vi "Save image.vi"(6 "Show filename dialog?":bool=TRUE, 7 "Extension (.tif)":string(combo)=".tif", 8 "error in":errorcluster, 9 "File name":string="image.tif", 10 "Image":T1, 11 "Base dir":path) -> (0 "error out":errorcluster, 3 "dup file":path)   [LabVIEW 2013, in "FileIO lib.lvlib"]
doc: "Creates a file and saves the current image. Image type is determined by the extension of the file name."
uses:
  FileIO lib.lvlib
  <vilib>/vision/Image Controls.llb/IMAQ Image.ctl
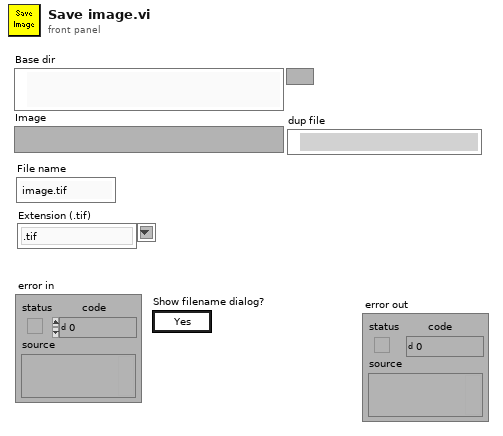
[diagram p1: front panel]
types:
  T1 = typedef "IMAQ Image.ctl" = refnum<image>
  T2 = enum32{"existing file", "new file", "new or existing file", "existing dir", "new dir", "new or existing dir", "existing file (use LLBs)", "new file (use LLBs)", "new or existing file (use LLBs)", "new or existing file or directory (use LLBs)"}
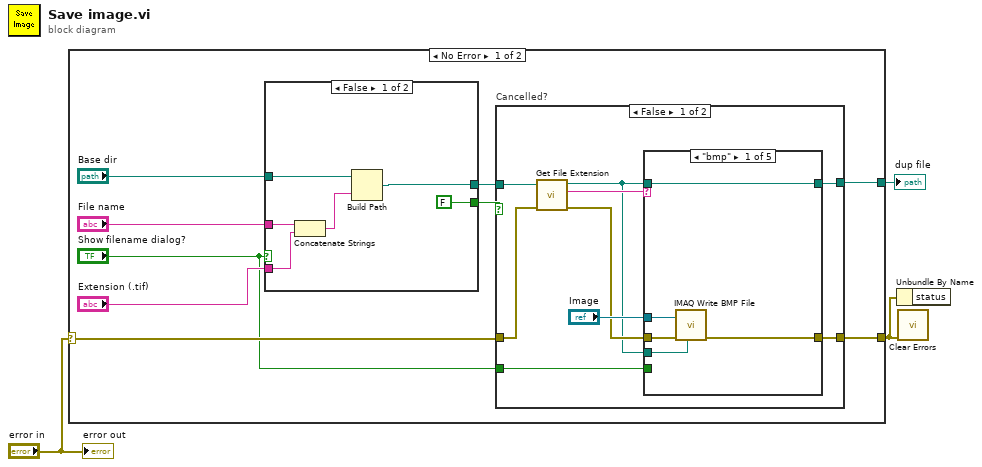
[diagram p0: block diagram]
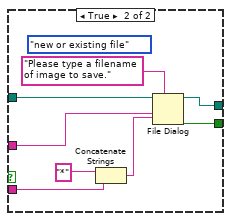
[diagram p2: hidden frame]
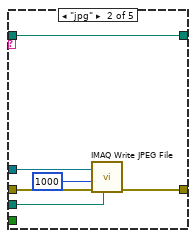
[diagram p3: hidden frame]
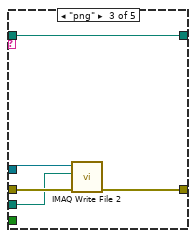
[diagram p4: hidden frame]
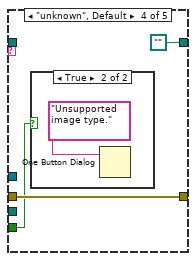
[diagram p5: hidden frame]
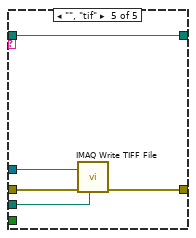
[diagram p7: hidden frame]
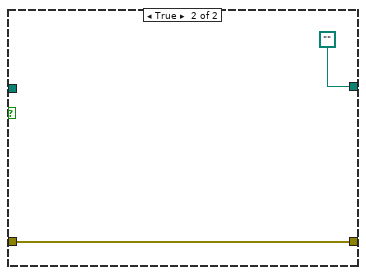
[diagram p8: hidden frame]
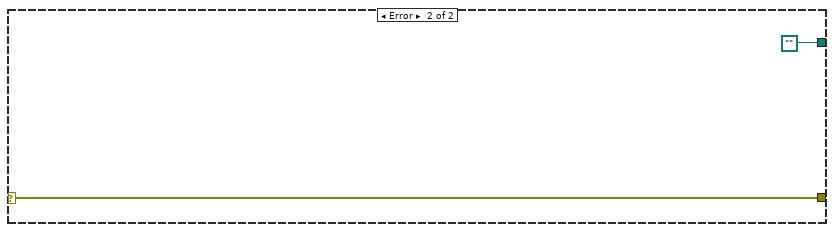
[diagram p9: hidden frame]
diagram:
  n1 = case shown="No Error" "error in" {
    selector: "error in" -> [w9 w64]
    tunnel: [w5 w64] -> w2
    tunnel: [w4 path ""] -> w1
    frame No Error {
      n2 = case shown="False" "Show filename dialog?" {
        tunnel: [w13 w26] -> w12
        tunnel: [FALSE ("cancelled") w25] -> w11
        tunnel: "Base dir" -> [w17 w23]
        tunnel: "File name" -> [w16 w22]
        tunnel: "Extension (.tif)" -> [w15 w20]
        frame False {
          n3 = Concatenate Strings(w16, w15) -> (w14:string)
          n4 = Build Path(base path=w17, name or relative path=w14) -> (appended path=w13:path)
        }
        frame True {
          (unwired) T2."new or existing file" ("select mode (2)")
          n5 = Concatenate Strings("*" ("pattern label"), w20) -> (w19:string)
          n6 = File Dialog(6:w19, 7:"Please type a filename of image to save." ("prompt"), 9:w22, 11:w23) -> (1:w25:bool, 3:w26:path)  [unwired: 1 in, 4 out]
        }
      }
      n7 = case "Cancelled?" shown="False" w11 {
        tunnel: w12 -> [w32 _]
        tunnel: w9 -> [w30 w62]
        tunnel: [w35 w62] -> w5
        tunnel: "Show filename dialog?" -> [w31 _]
        tunnel: [w27 path ""] -> w4
        frame False {
          n8 = call <vilib>:"Get File Extension.vi"("error in (no error)"=w30, "file"=w32) -> ("error out"=w29:errorcluster, "lowercase file extension"=w33:string, "dup file"=w28:path)  [unwired: 7 out]
          n9 = case shown="\"bmp\"" w33 {
            tunnel: w28 -> [w40 w46 w48 _ w57]
            tunnel: w29 -> [w38 w44 w49 w54 w59]
            tunnel: [w37 w43 w47 w54 w58] -> w35
            tunnel: "Image" -> [w39 w42 w50 _ w60]
            tunnel: w31 -> [_ _ _ w53 _]
            tunnel: w28 -> [w36 w41 w51 _ w56]
            tunnel: [w36 w41 w51 path "" w56] -> w27
            frame "bmp" {
              n10 = call "IMAQ Write BMP File"("error in (no error)"=w38, "File Path"=w40, "Image"=w39) -> ("error out"=w37:errorcluster)  [unwired: 2 in, 3 out]
            }
            frame "jpg" {
              n11 = call "IMAQ Write JPEG File"("error in (no error)"=w44, "Image Quality"=u32 1000, "File Path"=w46, "Image"=w42) -> ("error out"=w43:errorcluster)  [unwired: 1 in, 3 out]
            }
            frame "png" {
              n12 = call-poly "IMAQ Write File 2"("error in (no error)"=w49, "File Path"=w48, "Image"=w50) -> ("error out"=w47:errorcluster)  [unwired: 1 in, 7 out]
            }
            frame "unknown", Default {
              n13 = case shown="True" w53 {
                frame False {
                }
                frame True {
                  n14 = One Button Dialog(message="Unsupported image type.") -> ()  [unwired: 2 out]
                }
              }
            }
            frame "", "tif" {
              n15 = call "IMAQ Write TIFF File"("error in (no error)"=w59, "File Path"=w57, "Image"=w60) -> ("error out"=w58:errorcluster)  [unwired: 2 in, 3 out]
            }
          }
        }
        frame True {
        }
      }
    }
    frame Error {
    }
  }
  "dup file" <- w1
  n16 = Unbundle By Name(w2) -> ()  [unwired: 1 out]
  n17 = call <vilib>:"Clear Errors.vi"("error in (no error)"=w2) -> ()  [unwired: 7 out]
  "error out" <- "error in"
